vi "RemoteSession_CallCloseMeasurementLinkSessionWithDetach_RemoteSessionDetached.vi"(8 "error in (no error)":errorcluster) -> (0 "error out":errorcluster, 2 "result":string, 3 "pass":bool)   [LabVIEW 2020]
uses:
  Runtime/MeasurementLink niDCPower/Instrument/Instrument.lvclass
  Runtime/MeasurementLink Instrument/IInstrument/Close Session Behavior.ctl
  Runtime/MeasurementLink Instrument/IInstrument/IInstrument.lvclass
  MeasurementServerTests.lvlib
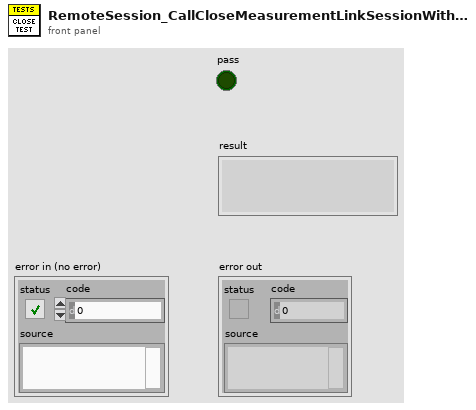
[diagram p1: front panel]
types:
  T1 = typedef "MeasurementLink Instrument.lvlib/IInstrument.lvclass/Close Session Behavior.ctl" = enum16{"Close Session", "Detach Session"}
  T2 = typedef "MeasurementLink Instrument.lvlib/IInstrument.lvclass/Remote Connection Options.ctl" = cluster{"session name":string, "address":string, "port":u32}
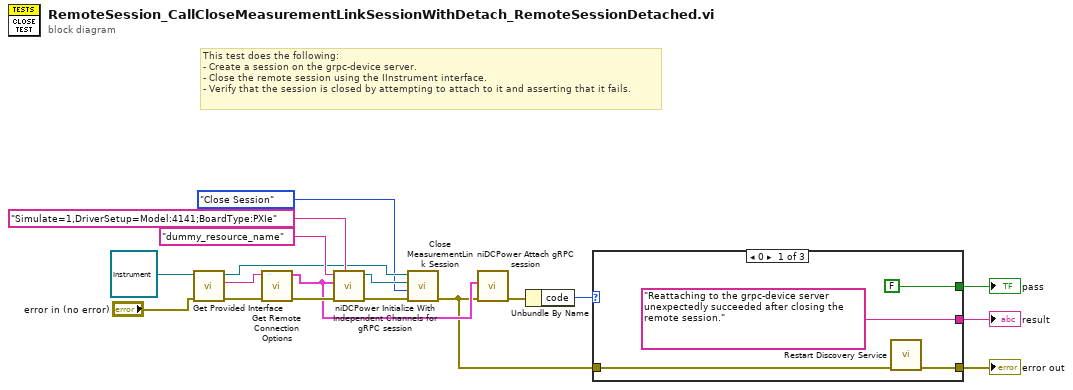
[diagram p0: block diagram]
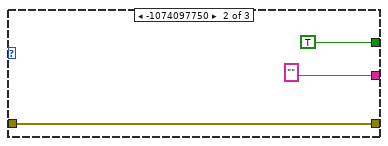
[diagram p2: hidden frame]
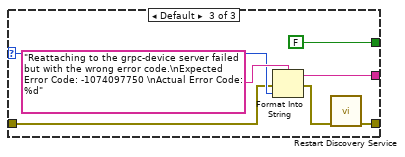
[diagram p3: hidden frame]
diagram:
  # "This test does the following:\n- Create a session on the grpc-device server.\n- Close the remote session using the IInstrument interface.\n- Verify that the session is closed by attempting to attach to it and asserting that it fails."
  n1 = call-dynamic "Get Provided Interface.vi"("error in (no error)"="error in (no error)", "instrument in"=refnum<class "Instrument.lvclass"> refnum ("MeasurementLink niDCPower.lvlib:Instrument.lvclass")) -> ("error out"=w15:errorcluster, "provided interface"=w14:string, "instrument out"=w11:refnum<class "Instrument.lvclass">)  [unwired: 7 in]
  n2 = call "Get Remote Connection Options.vi"("error in (no error)"=w15, "provided interface"=w14) -> ("error out"=w17:errorcluster, "remote connection options"=w8:T2)  [unwired: 8 in]
  n3 = call <instrlib>:"niDCPower Initialize With Independent Channels for gRPC session.vi"("option string"="Simulate=1,DriverSetup=Model:4141;BoardType:PXIe", "error in (no error)"=w17, "gRPC options"=w8, "resource name"="dummy_resource_name") -> ("error out"=w12:errorcluster, "instrument handle out"=w10:refnum<k15>)  [unwired: 6 in]
  n4 = call-dynamic "Close MeasurementLink Session.vi"("error in (no error)"=w12, "close session behavior"=Close_Session_Behavior."Close Session", "session in"=w10, "instrument in"=w11) -> ("error out"=w2:errorcluster)  [unwired: 7 in]
  n5 = call <instrlib>:"niDCPower Attach gRPC session.vi"("error in (no error)"=w2, "gRPC options"=w8) -> ("error out"=w7:errorcluster)  [unwired: 8 in, 1 out]
  n6 = Unbundle By Name(w7) -> ("code"=w5:i32)
  n7 = case shown="0" w5 {
    selector: w5 -> [_ _ w31]
    tunnel: ["Reattaching to the grpc-device server unexpectedly succeeded after closing the remote session." ("f") "" ("f") w30] -> w3
    tunnel: [FALSE TRUE FALSE] -> w4
    tunnel: w2 -> [w20 w23 w28]
    tunnel: [w19 w23 w26] -> w1
    frame 0 {
      n8 = call "Restart Discovery Service.vi"("error in"=w20) -> ("error out"=w19:errorcluster)  [unwired: 10 in]
    }
    frame -1074097750 {
    }
    frame Default {
      n9 = Format Into String(format string="Reattaching to the grpc-device server failed but with the wrong error code.\nExpected Error Code: -1074097750 \nActual Error Code: %d" ("f"), error in=w28, w31) -> (resulting string=w30:string, error out=w27:errorcluster)  [unwired: 1 in]
      n10 = call "Restart Discovery Service.vi"("error in"=w27) -> ("error out"=w26:errorcluster)  [unwired: 10 in]
    }
  }
  "error out" <- w1
  "pass" <- w4
  "result" <- w3
